vi "CreateTxtFile.vi"(11 "pathIn":path=path "C:/Users/Robotics/Desktop/AutonInfo") -> (3 "refnumOut":refnum<file>)   [LabVIEW 2017]
panel:
  out "pathOut":path
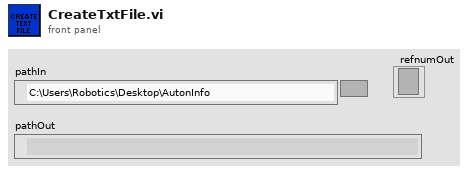
[diagram p1: front panel]
types:
  T1 = enum16{"open", "replace", "create", "open or create", "replace or create", "replace or create with confirmation"}
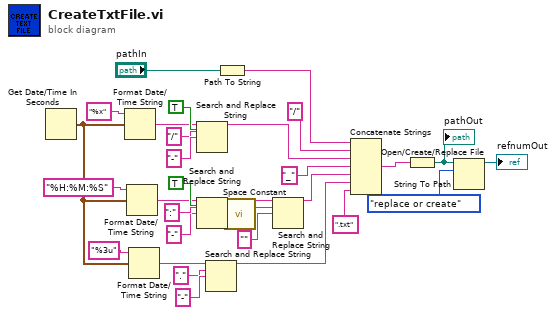
[diagram p0: block diagram]
diagram:
  n1 = Get Date/Time In Seconds() -> (seconds since 1Jan1904=w6:timestamp)
  n2 = Format Date/Time String(time format string (%c)="%x", seconds (now)=w6) -> (date/time string=w25:string)  [unwired: 1 in]
  n3 = Format Date/Time String(time format string (%c)="%H:%M:%S", seconds (now)=w6) -> (date/time string=w22:string)  [unwired: 1 in]
  n4 = Format Date/Time String(time format string (%c)="%3u", seconds (now)=w6) -> (date/time string=w2:string)  [unwired: 1 in]
  n5 = Search and Replace String(replace all?=TRUE ("replace all? (F)"), input string=w25, search string="/", replace string="-" ("replace string (\"\")")) -> (result string=w18:string)  [unwired: 4 in, 3 out]
  n6 = Search and Replace String(replace all?=TRUE ("replace all? (F)"), input string=w22, search string=":", replace string="-" ("replace string (\"\")")) -> (result string=w14:string)  [unwired: 4 in, 3 out]
  n7 = Search and Replace String(input string=w2, search string=".", replace string="-" ("replace string (\"\")")) -> (result string=w1:string)  [unwired: 5 in, 3 out]
  n8 = Path To String(path="pathIn") -> (string=w16:string)
  n9 = call <vilib>:"Space Constant.vi"() -> ("String"=w11:string)
  n10 = Search and Replace String(input string=w14, search string=w11, replace string="" ("search string")) -> (result string=w12:string)  [unwired: 5 in, 3 out]
  n11 = Concatenate Strings(w16, "/" ("string"), w18, "_" ("string"), w12, w1, ".txt" ("string")) -> (w17:string)
  n12 = String To Path(string=w17) -> (path=w10:path)
  "pathOut" <- w10
  n13 = Open/Create/Replace File(file path (use dialog)=w10, operation (0:open)=T1."replace or create") -> (refnum out=→"refnumOut":refnum<file>)  [unwired: 4 in, 2 out]
